vi "Insert Table.vi"(7 "Location":T1={"Sheet Name"="", "Name"="", "Display Name"="", "Range or Cell Address"="A1:B2"}, 8 "error in":errorcluster, 9 "Cell Values":variant[][](array[variant]), 10 "Header Names":string[](array[string]), 11 "SpreadsheetDoc in":refnum<k24>) -> (0 "error out":errorcluster, 3 "SpreadsheetDoc out":refnum<k24>)   [LabVIEW 2019, in "Open Xml.lvlib"]
doc: "Inserts a structured table"
uses:
  Open Xml.lvlib
  D:/git/Open-Xml-LabVIEW/Source/DocumentFormat.OpenXml.dll
  DocumentFormat.OpenXml.dll
  D:/git/Open-Xml-LabVIEW/Source/DocumentFormat.OpenXml.Framework.dll
  DocumentFormat.OpenXml.Framework.dll
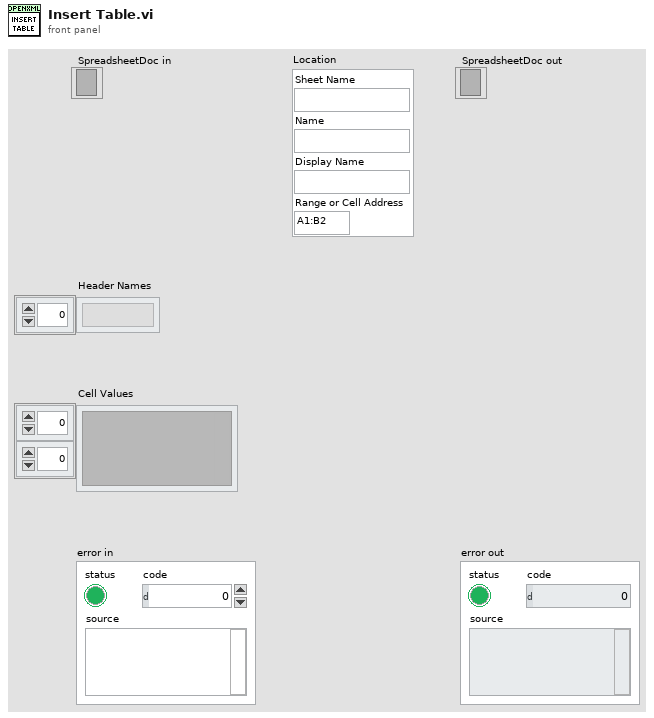
[diagram p1: front panel]
types:
  T1 = cluster{"Sheet Name":string, "Name":string, "Display Name":string, "Range or Cell Address":string}
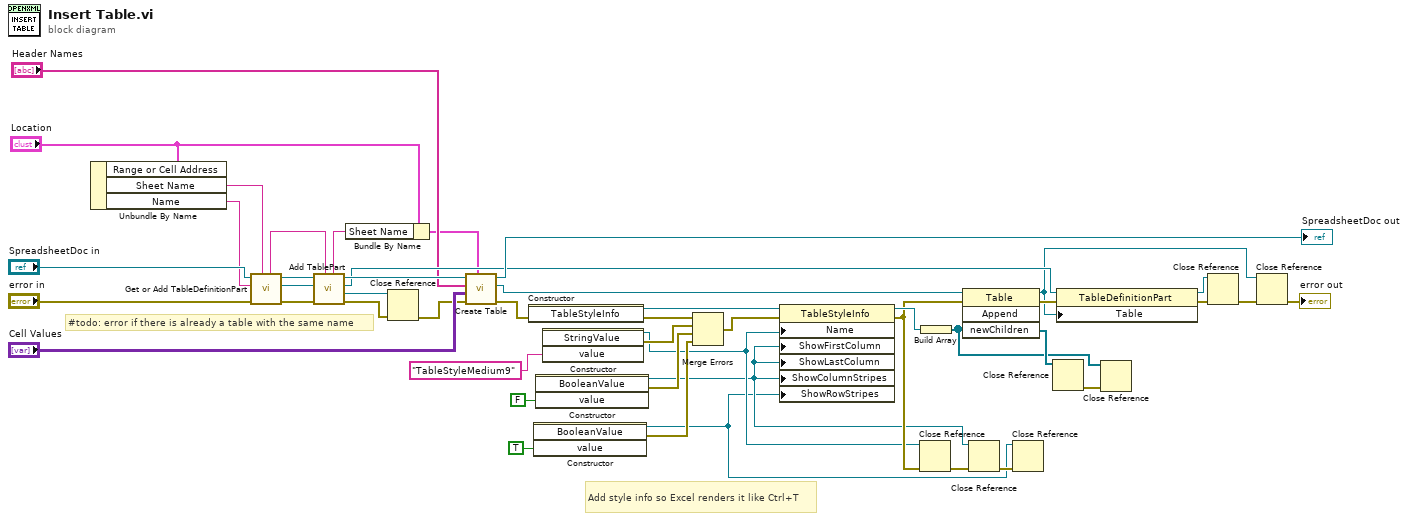
[diagram p0: block diagram]
diagram:
  # "Add style info so Excel renders it like Ctrl+T"
  # "#todo: error if there is already a table with the same name"
  n1 = Unbundle By Name("Location") -> ("Sheet Name"=w43:string, "Name"=w44:string)  [unwired: 1 out]
  n2 = call "Get or Add TableDefinitionPart.vi"("Sheet Name"=w43, "error in"="error in", "Table Name"=w44, "SpreadsheetDoc in"="SpreadsheetDoc in") -> ("error out"=w36:errorcluster, "TableDefinitionPart"=w38:refnum<k24>, "SpreadsheetDo out"=w42:refnum<k24>, "Sheet Name"=w41:string)  [unwired: 4 in]
  n3 = call "Add TablePart.vi"("Sheet Name"=w41, "error in"=w36, "TableDefinitionPart in"=w38, "SpreadsheetDoc in"=w42) -> ("error out"=w10:errorcluster, "TablePart"=w11:refnum<k24>, "TableDefinitionPart out"=w35:refnum<k24>, "SpreadsheetDoc out"=w40:refnum<k24>, "Sheet Name"=w31:string)  [unwired: 3 in]
  n4 = Bundle By Name(cluster="Location", "Sheet Name"=w31) -> (w32:T1)
  n5 = Close Reference(reference=w11, error in (no error)=w10) -> (error out=w9:errorcluster)
  n6 = call "Create Table.vi"("Location"=w32, "error in"=w9, "Values"="Cell Values", "Header Names"="Header Names", "SpreadsheetDoc in"=w40) -> ("error out"=w24:errorcluster, "Table"=w25:refnum<k24>, "SpreadsheetDoc out"=→"SpreadsheetDoc out":refnum<k24>)  [unwired: 4 in]
  n7 = constructor class="TableStyleInfo"(error in=w24) -> (reference out=w27:refnum<k24>, error out=w28:errorcluster)  [unwired: 2 in, 1 out]
  n8 = constructor class="BooleanValue"("value"=TRUE) -> (reference out=w3:refnum<k24>, error out=w19:errorcluster)  [unwired: 3 in, 2 out]
  n9 = constructor class="BooleanValue"("value"=FALSE) -> (reference out=w5:refnum<k24>, error out=w18:errorcluster)  [unwired: 3 in, 2 out]
  n10 = constructor class="StringValue"("value"="TableStyleMedium9") -> (reference out=w7:refnum<k24>, error out=w17:errorcluster)  [unwired: 3 in, 2 out]
  n11 = Merge Errors(w28, w17, w18, w19) -> (w20:errorcluster)
  n12 = property class="TableStyleInfo"(reference=w27, error in=w20, "Name"=w7, "ShowFirstColumn"=w5, "ShowLastColumn"=w5, "ShowColumnStripes"=w5, "ShowRowStripes"=w3) -> (reference out=w23:refnum<k24>, error out=w8:errorcluster)
  n13 = Close Reference(reference=w7, error in (no error)=w8) -> (error out=w6:errorcluster)
  n14 = Build Array(w23) -> (w1:refnum<k24>[])
  n15 = invoke class="Table" method="Append"(reference=w25, error in=w8, "newChildren"=w1) -> (reference out=w12:refnum<k24>, error out=w26:errorcluster, "newChildren"=w14:refnum<k24>[])  [unwired: 1 in, 1 out]
  n16 = Close Reference(reference=w5, error in (no error)=w6) -> (error out=w4:errorcluster)
  n17 = Close Reference(reference=w3, error in (no error)=w4) -> ()  [unwired: 1 out]
  n18 = Close Reference(reference=w14) -> (error out=w2:errorcluster)  [unwired: 1 in]
  n19 = property class="TableDefinitionPart"(reference=w35, error in=w26, "Table"=w12) -> (reference out=w29:refnum<k24>, error out=w39:errorcluster)
  n20 = Close Reference(reference=w1, error in (no error)=w2) -> ()  [unwired: 1 out]
  n21 = Close Reference(reference=w29, error in (no error)=w39) -> (error out=w30:errorcluster)
  n22 = Close Reference(reference=w12, error in (no error)=w30) -> (error out=→"error out":errorcluster)
